vi "Add Timestamp.vi"(8 "error in (no error)":errorcluster, 9 "Counter Value":u32, 10 "Channel":i32, 11 "TimeStamper in":refnum<class "TimeStamper.lvclass">) -> (0 "error out":errorcluster, 2 "Timestamp":T1, 3 "TimeStamper out":refnum<class "TimeStamper.lvclass">)   [LabVIEW 2010, in "TimeStamper.lvclass"]
uses:
  TimeStamper.lvclass
  TimeStamper.lvclass/TimeStamper.ctl
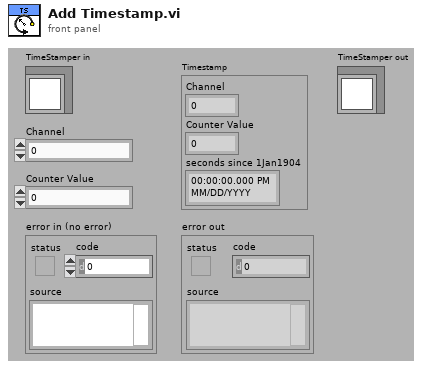
[diagram p1: front panel]
types:
  T1 = cluster{"Channel":i32, "Counter Value":u32, "seconds since 1Jan1904":timestamp}
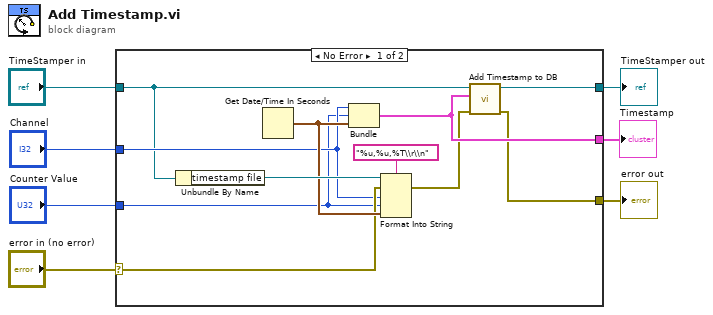
[diagram p0: block diagram]
diagram:
  n1 = case shown="No Error" "error in (no error)" {
    selector: "error in (no error)" -> [w15 w20]
    tunnel: [w8 w20] -> w6
    tunnel: [w11 w19] -> w4
    tunnel: "TimeStamper in" -> [w12 w19]
    tunnel: "Channel" -> [w14 _]
    tunnel: "Counter Value" -> [w13 _]
    tunnel: [w10 _] -> w1
    frame No Error {
      n2 = Unbundle By Name(w12) -> ("timestamp file"=w18:refnum<file>)
      n3 = Get Date/Time In Seconds() -> (seconds since 1Jan1904=w16:timestamp)
      n4 = Bundle("Channel"=w14, "Counter Value"=w13, "seconds since 1Jan1904"=w16) -> (w10:T1)  [unwired: 1 in]
      n5 = Format Into String(format string="%u,%u,%T\\r\\n", initial string=w18, error in=w15, w14, w13, w16) -> (error out=w9:errorcluster)  [unwired: 1 out]
      n6 = call-dynamic "Add Timestamp to DB.vi"("error in (no error)"=w9, "Timestamp"=w10, "TimeStamper in"=w12) -> ("error out"=w8:errorcluster, "TimeStamper out"=w11:refnum<class "TimeStamper.lvclass">)  [unwired: 7 in]
    }
    frame Error {
    }
  }
  "error out" <- w6
  "TimeStamper out" <- w4
  "Timestamp" <- w1
